vi "Single Z Ramp Approach.vi"(0 "Experimental Queue":T1) -> ()   [LabVIEW 2013]
uses:
  Runtime/Runtime Queue.ctl
  Runtime/Experimental Configuration.ctl
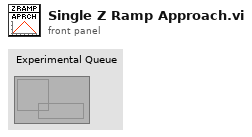
[diagram p1: front panel]
types:
  T1 = typedef "Runtime Queue.ctl" = refnum<queue>
  T2 = cluster{"Output Waveforms":waveform(dbl)[], "Output Channels":string, "Input Channels":string, "occurrence":refnum<k4>}
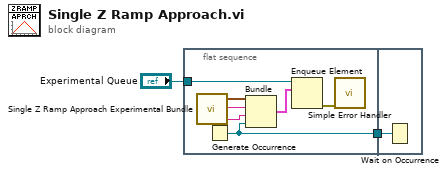
[diagram p0: block diagram]
diagram:
  n1 = flat-sequence {
    tunnel: [w3] -> w2
    tunnel: "Experimental Queue" -> [w9]
    tunnel: w2 -> [w10]
    frame #0 {
      n2 = call "Single Z Ramp Approach Experimental Bundle.vi"() -> ("Input Channels"=w6:string, "Output Channels"=w7:string, "Output Waveforms"=w8:waveform(dbl)[])
      n3 = Generate Occurrence() -> (w3:refnum<k4>)
      n4 = Bundle("Output Waveforms"=w8, "Output Channels"=w7, "Input Channels"=w6, "occurrence"=w3) -> (w5:T2)  [unwired: 1 in]
      n5 = Enqueue Element(queue=w9, element=w5) -> (error out=w4:errorcluster)  [unwired: 2 in, 2 out]
      n6 = call <vilib>:"Simple Error Handler.vi"("error in (no error)"=w4) -> ()  [unwired: 4 in, 5 out]
    }
    frame #1 {
      n7 = Wait on Occurrence(2:w10) -> ()  [unwired: 2 in, 1 out]
    }
  }
